vi "add 6221-2182-DC initalize(SubVI).vi"(9 "字符串":string, 10 "model":string="Delta") -> (0 "连接的字符串":string, 3 "ok or cancel":bool=TRUE)   [LabVIEW 2019, in "Add Seq.lvlib"]
uses:
  Add Seq.lvlib
  lib/Keithley 622x/Configure/Source/Typedefs/KE622x -- Current Range.ctl
  lib/Keithley 622x/Configure/Source/Typedefs/KE622x -- Current Ranges.ctl
  lib/Keithley 622x/Typedefs/KE622x -- On Off Control.ctl
  lib/Keithley 622x/Configure/Output/Typedefs/KE6221 -- Output Response.ctl
  lib/Keithley 622x/Configure/Source/Typedefs/KE622x -- Current Level.ctl
  lib/Keithley 622x/Configure/Source/Typedefs/KE622x -- Voltage Limit.ctl
  lib/Keithley 622x/Configure/2182 -A/Low Level/Typedefs/KE2182 -- Voltage Ranges.ctl
  lib/Keithley 622x/Configure/2182 -A/Low Level/Typedefs/KE2182 -- Filter Type.ctl
  lib/Keithley 622x/Configure/2182 -A/Low Level/Typedefs/KE2182 -- Filter Count.ctl
  lib/Keithley 622x/Configure/2182 -A/Low Level/Typedefs/KE2182 -- Filter Window.ctl
  lib/Keithley 622x/Configure/2182 -A/Low Level/Typedefs/KE2182 -- NPLCs.ctl
  SubVI.lvlib
  lib/Keithley 622x/Keithley 622x.lvlib
panel:
  in  "2812 -A Params In":T6={"Auto Range?"=TRUE, "Man / Selected\nRange"=enum."10mV", "Enable Digital\nFilter?"=FALSE, "Filter Type"=enum."Moving", "Filter Count"=10, "Filter\nWindow (%)"=0.01, "Enable Analog\nFilter?"=FALSE, "NPLCs"=5} {"Filter\nWindow (%)" min=0.0 max=10.0 step=0.01 format="%.2f"; "Filter Count" min=1 max=100; "NPLCs" min=1 max=10}
  in  "Turn Off Output If Voltage Limit?":bool=TRUE
  in  "Voltage Limit (V)":T7=10.0 min=0.1 max=105.0 step=0.01 format="%.2p"
  in  "Current Level (A)":T8=0.001 min=-0.105 max=0.105 format="%.4p"
  in  "Output Response":T9=enum."Slow"
  in  "Analog Filter State":T10
  in  "Current Range In":T11={"Auto Range?"=TRUE, "Man / Selected\nRange"=enum."2nA"}
  out "错误输出":errorcluster
  in  "load":bool
  in  "cancel":bool
  in  "ok":bool
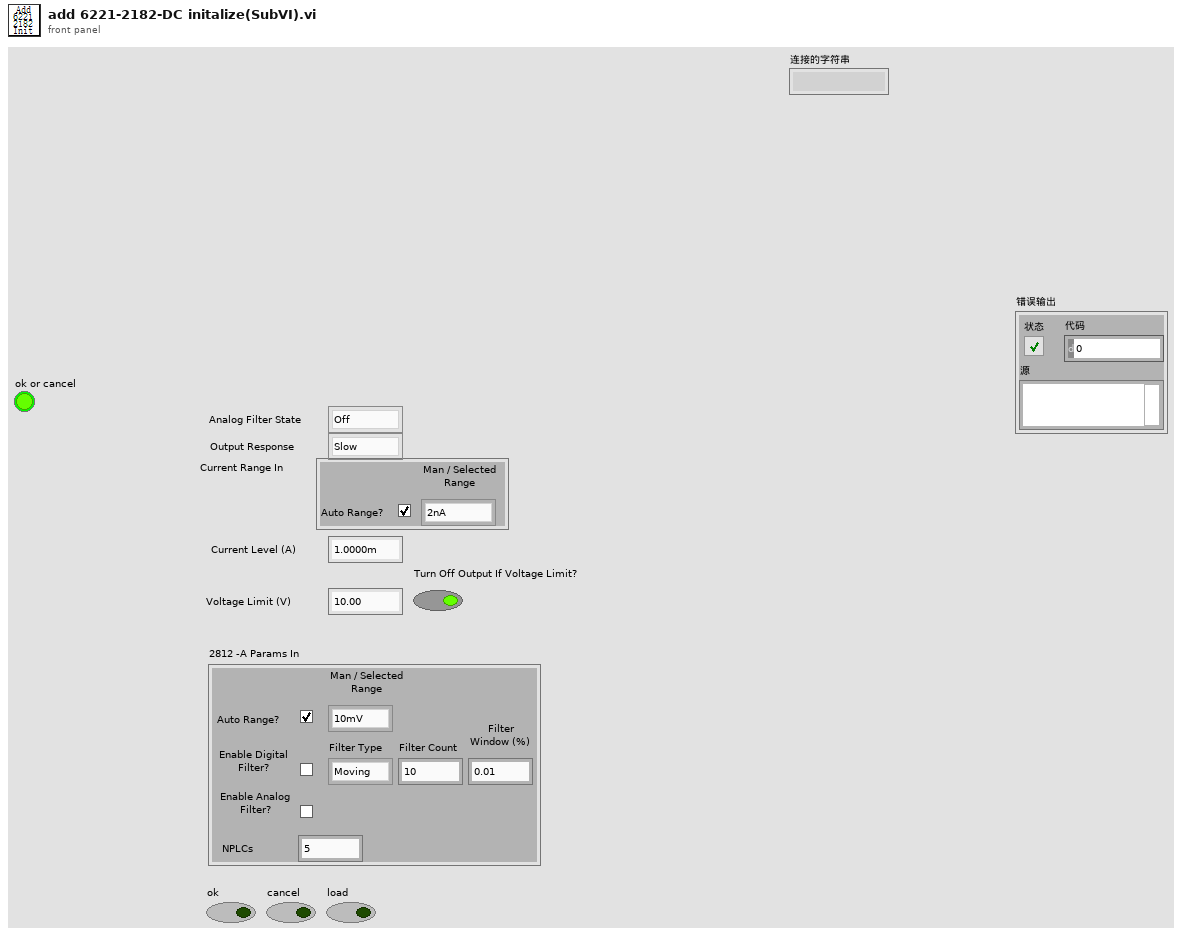
[diagram p1: front panel]
types:
  T1 = typedef "Keithley 622x.lvlib/KE2182 -- Voltage Ranges.ctl" = enum16{"10mV", "100mV", "1V", "10V", "100V"}
  T2 = typedef "Keithley 622x.lvlib/KE2182 -- Filter Type.ctl" = enum16{"Moving", "Repeat"}
  T3 = typedef "Keithley 622x.lvlib/KE2182 -- Filter Count.ctl" = u32
  T4 = typedef "Keithley 622x.lvlib/KE2182 -- Filter Window.ctl" = dbl
  T5 = typedef "Keithley 622x.lvlib/KE2182 -- NPLCs.ctl" = u32
  T6 = cluster{"Auto Range?":bool, "Man / Selected\nRange":T1, "Enable Digital\nFilter?":bool, "Filter Type":T2, "Filter Count":T3, "Filter\nWindow (%)":T4, "Enable Analog\nFilter?":bool, "NPLCs":T5}
  T7 = typedef "Keithley 622x.lvlib/KE622x -- Voltage Limit.ctl" = dbl
  T8 = typedef "Keithley 622x.lvlib/KE622x -- Current Level.ctl" = dbl
  T9 = typedef "Keithley 622x.lvlib/KE6221 -- Output Response.ctl" = enum16{"Fast", "Slow"}
  T10 = typedef "Keithley 622x.lvlib/KE622x -- On Off Control.ctl" = enum16{"Off", "On"}
  T11 = typedef "Keithley 622x.lvlib/KE622x -- Current Range.ctl" = cluster{"Auto Range?":bool, "Man / Selected\nRange":T12}
  T12 = typedef "Keithley 622x.lvlib/KE622x -- Current Ranges.ctl" = enum16{"2nA", "20nA", "200nA", "2uA", "20uA", "200uA", "2mA", "20mA", "100mA"}
  T13 = enum16{"open", "replace", "create", "open or create", "replace or create"}
  T14 = enum16{"open", "replace", "create", "open or create", "replace or create", "replace or create with confirmation"}
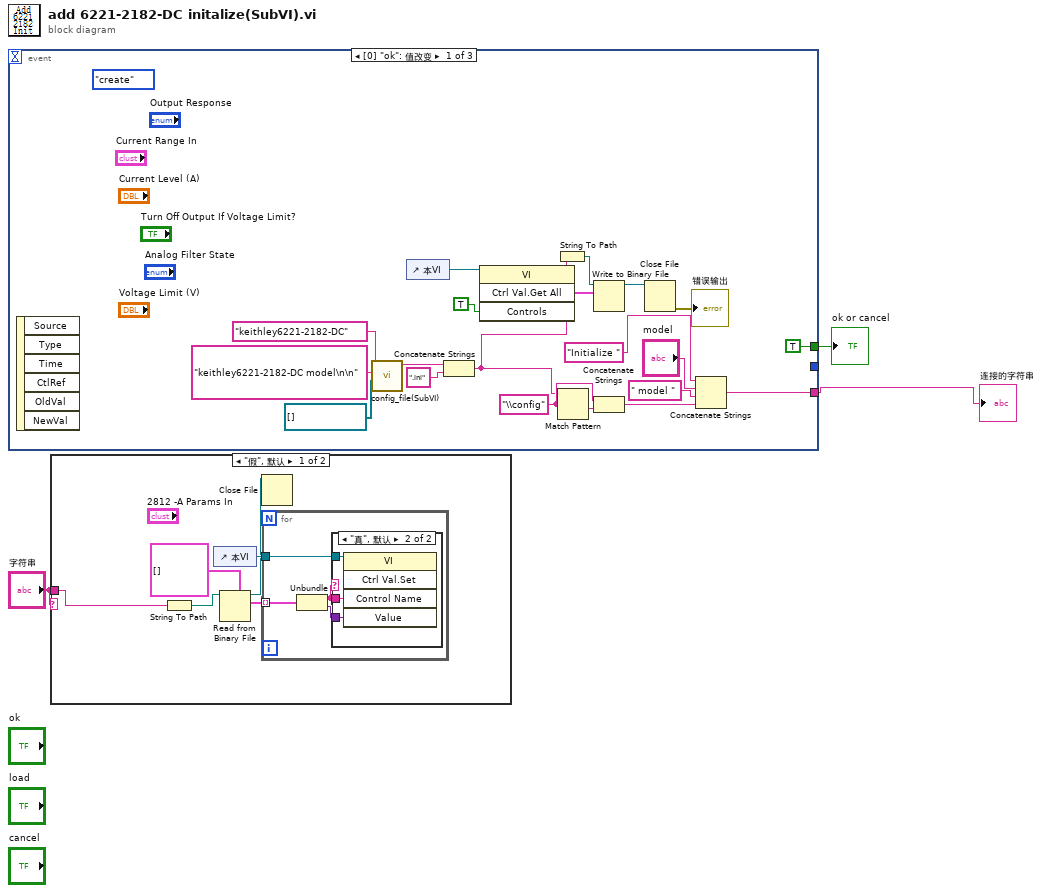
[diagram p0: block diagram]
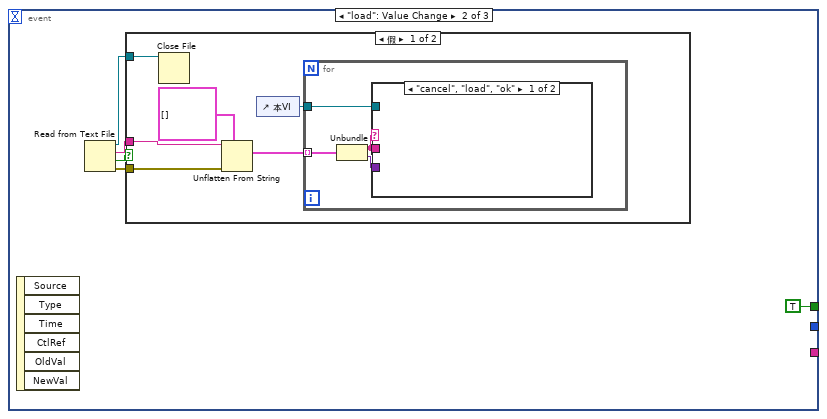
[diagram p4: hidden frame]
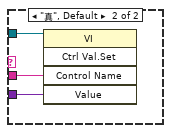
[diagram p5: hidden frame]
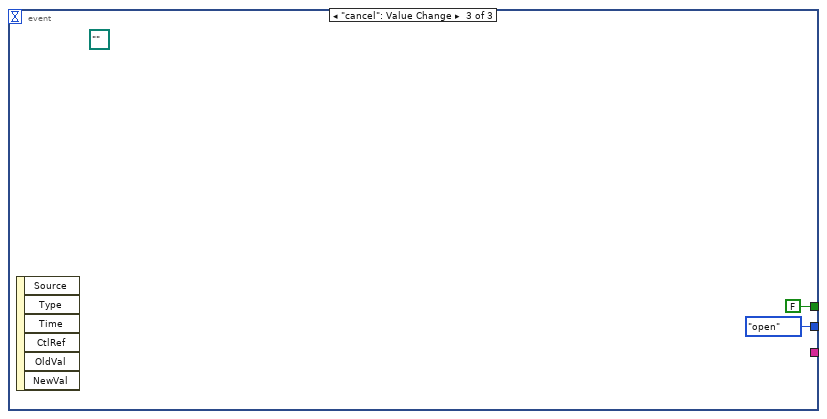
[diagram p7: hidden frame]
diagram:
  n1 = event shown="[0] \"ok\": 值改变" {
    selector: _ -> [_ _ _]
    dyn-events: _ -> [_ _ _]
    timeout: _ -> [_ _ _]
    tunnel: [_ _ T13."open" ("operation(0:open)")] -> _
    tunnel: [TRUE TRUE FALSE] -> w3
    tunnel: [w12 _ _] -> w1
    event "ok": Value Change {
      w7 = "\\config" ("正则表达式")
      (unwired) T14."create" ("操作(0:open)")
      n2 = event-data() -> ()  [unwired: 1 in, 6 out]
      n3 = call "config_file(SubVI).vi"("all ref"=refnum<vi>[] [], "文件抬头"="keithley6221-2182-DC model\n\n", "文件夹名称"="keithley6221-2182-DC" ("字符串")) -> ("字符串输出"=w17:string)  [unwired: 8 in]
      n4 = control-ref of="本VI"() -> (w20:refnum<vi>)
      n5 = Concatenate Strings(w17, ".ini" ("字符串")) -> (w5:string)
      n6 = invoke class="VI" method="Ctrl Val.Get All"(reference=w20, "Controls"=TRUE ("控件")) -> ("Get All Control Values Variant"=w10:cluster{"Name":string, "Variant Data":variant}[])  [unwired: 2 in, 3 out]
      n7 = String To Path(string=w5) -> (path=w11:path)
      n8 = Match Pattern(string=w5, regular expression=w7) -> (after substring=w6:string)  [unwired: 1 in, 3 out]
      n9 = Write to Binary File(file (use dialog)=w11, data=w10) -> (refnum out=w9:refnum<file>)  [unwired: 4 in, 2 out]
      n10 = Concatenate Strings(w7, w6) -> (w4:string)
      n11 = Close File(refnum=w9) -> (error out=→"错误输出":errorcluster)  [unwired: 1 in, 1 out]
      n12 = Concatenate Strings("Initialize " ("字符串"), "model", " model " ("字符串"), w4) -> (w12:string)
    }
    event "load": Value Change {
      n13 = event-data() -> ()  [unwired: 1 in, 6 out]
      n14 = Read from Text File() -> (refnum out=w27:refnum<file>, text=w25:string, cancelled=w24:bool, error out=w26:errorcluster)  [unwired: 4 in]
      n15 = case shown="假" w24 {
        tunnel: w27 -> [w34 _]
        tunnel: w26 -> [w32 _]
        tunnel: w25 -> [w31 _]
        frame False {
          n16 = Close File(refnum=w34) -> ()  [unwired: 1 in, 2 out]
          n17 = Unflatten From String(type=cluster{"Name":string, "Variant Data":variant}[] [] ("控件值:获取全部"), binary string=w31, error in (no error)=w32) -> (value=w30:cluster{"Name":string, "Variant Data":variant}[])  [unwired: 2 in, 2 out]
          n18 = control-ref of="本VI"() -> (w29:refnum<vi>)
          n19 = for {
            tunnel: w30 -> [w38] mode=indexing
            tunnel: w29 -> [w37]
            n20 = Unbundle(w38) -> ("Name"=w35:string, "Variant Data"=w36:variant)
            n21 = case shown="\"cancel\", \"load\", \"ok\"" w35 {
              tunnel: w37 -> [_ w41]
              tunnel: w35 -> [_ w40]
              tunnel: w36 -> [_ w39]
              frame "cancel", "load", "ok" {
              }
              frame "真", Default {
                n22 = invoke class="VI" method="Ctrl Val.Set"(reference=w41, "Control Name"=w40, "Value"=w39) -> ()  [unwired: 2 in, 5 out]
              }
            }
          }
        }
        frame True {
        }
      }
    }
    event "cancel": Value Change {
      (unwired) path "" ("path")
      n23 = event-data() -> ()  [unwired: 1 in, 6 out]
    }
  }
  "ok or cancel" <- w3
  "连接的字符串" <- w1
  n24 = case shown="\"假\", 默认" "字符串" {
    tunnel: "字符串" -> [w49 _]
    frame "假", Default {
      n25 = String To Path(string=w49) -> (path=w47:path)
      n26 = control-ref of="本VI"() -> (w48:refnum<vi>)
      n27 = Read from Binary File(5:cluster{"Name":string, "Variant Data":variant}[] [] ("控件值:获取全部"), 11:w47) -> (2:w45:cluster{"Name":string, "Variant Data":variant}[], 3:w44:refnum<file>)  [unwired: 4 in, 2 out]
      n28 = Close File(refnum=w44) -> ()  [unwired: 1 in, 2 out]
      n29 = for {
        tunnel: w45 -> [w53] mode=indexing
        tunnel: w48 -> [w52]
        n30 = Unbundle(w53) -> ("Name"=w50:string, "Variant Data"=w51:variant)
        n31 = case shown="\"真\", 默认" w50 {
          tunnel: w52 -> [_ w56]
          tunnel: w50 -> [_ w55]
          tunnel: w51 -> [_ w54]
          frame "cancel", "load", "ok" {
          }
          frame "真", Default {
            n32 = invoke class="VI" method="Ctrl Val.Set"(reference=w56, "Control Name"=w55, "Value"=w54) -> ()  [unwired: 2 in, 5 out]
          }
        }
      }
    }
    frame "" {
    }
  }
